vi "Menue_Event.vi"(4 "Menue 2":refnum<user-event>, 5 "Event Data":cluster{"sender":refnum<k24>, "e":refnum<k24>}, 6 "Control Ref":refnum<k24>, 7 "Event Common Data":T1) -> ()   [LabVIEW 2016, in "MenueItem.lvclass"]
uses:
  MenueItem.lvclass
  System.Windows.Forms
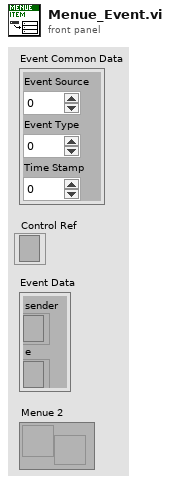
[diagram p1: front panel]
types:
  T1 = cluster{"Event Source":i32, "Event Type":u32, "Time Stamp":u32}
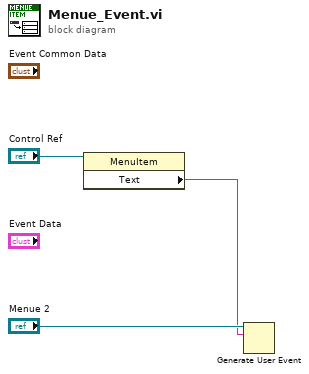
[diagram p0: block diagram]
diagram:
  n1 = property class="MenuItem"(reference="Control Ref") -> ("Text"=w1:string)  [unwired: 1 in, 2 out]
  n2 = Generate User Event(user event="Menue 2", event data cluster=w1) -> ()  [unwired: 2 in, 2 out]
